vi "Example_unloadSlot.vi"() -> ()   [LabVIEW 2021, in "BrainStem2_LabVIEW_Library.lvlib"]
uses:
  BrainStem2_LabVIEW_Library.lvlib
panel:
  out "Array - Numeric":u8[](array[numeric])
  out "Error":dbl
  out "Unloaded Length":dbl
  out "Slot Capacity":dbl
  in  "Slot":dbl
  in  "Store":dbl
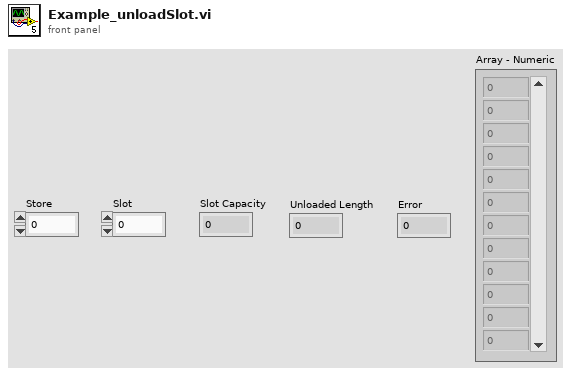
[diagram p1: front panel]
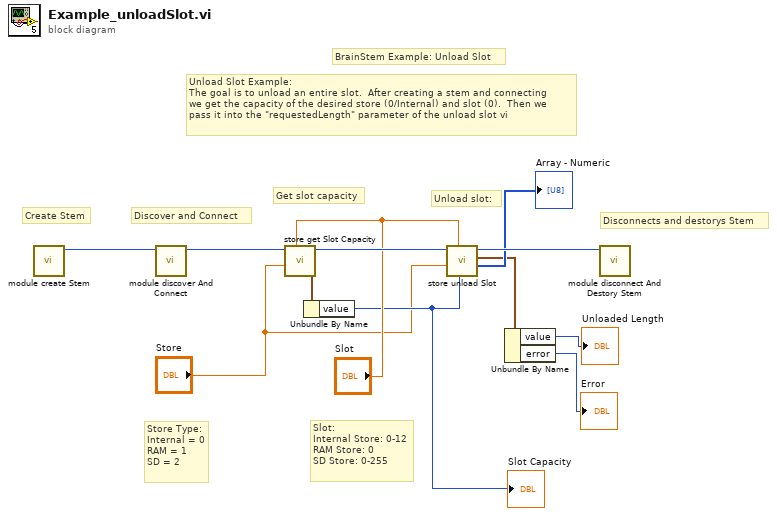
[diagram p0: block diagram]
diagram:
  # "Store Type:\nInternal = 0\nRAM = 1\nSD = 2"
  # "Slot:\nInternal Store: 0-12\nRAM Store: 0\nSD Store: 0-255"
  # "BrainStem Example: Unload Slot"
  # "Unload Slot Example:\nThe goal is to unload an entire slot.  After creating a stem and connecting\nwe get the capacity of the desired store (0/Internal) and slot (0).  Then we\npass it into the \"requestedLength\" parameter of the unload slot vi"
  # "Disconnects and destorys Stem"
  # "Unload slot:"
  # "Get slot capacity"
  # "Discover and Connect"
  # "Create Stem"
  n1 = call "module create Stem.vi"() -> ("id out"=w12:u32)  [unwired: 9 in, 2 out]
  n2 = call "module discover And Connect.vi"("id"=w12) -> ("id out"=w11:u32)  [unwired: 8 in, 2 out]
  n3 = call "store get Slot Capacity.vi"("slot"="Slot", "index"="Store", "id"=w11) -> ("result out"=w7:cluster{"value":i32, "error":i32}, "id out"=w10:u32)  [unwired: 6 in, 1 out]
  n4 = Unbundle By Name(w7) -> ("value"=w6:i32)
  "Slot Capacity" <- w6
  n5 = call "store unload Slot.vi"("bufferLength"=w6, "slot"="Slot", "index"="Store", "id"=w10) -> ("buffer"=→"Array - Numeric":u8[], "result out"=w3:cluster{"value":i32, "error":i32}, "id out"=w9:u32)  [unwired: 4 in, 1 out]
  n6 = Unbundle By Name(w3) -> ("value"=→"Unloaded Length":i32, "error"=→"Error":i32)
  n7 = call "module disconnect And Destory Stem.vi"("id"=w9) -> ()  [unwired: 8 in, 3 out]
